vi "Initialize.vi"(8 "error in (no error)":errorcluster, 9 "Requestor":string, 10 "Requestee":string, 11 "RUS Measurement in":refnum<class "RUS Measurement.lvclass">) -> (0 "error out":errorcluster, 3 "RUS Measurement out":refnum<class "RUS Measurement.lvclass">)   [LabVIEW 2015, in "RUS Measurement.lvclass"]
uses:
  RUS Measurement.lvclass
  RUS Measurement.lvclass/RUS Measurement.ctl
  Write Active.vi
  Mag Lab Measurement/Mag Lab Measurement.lvclass
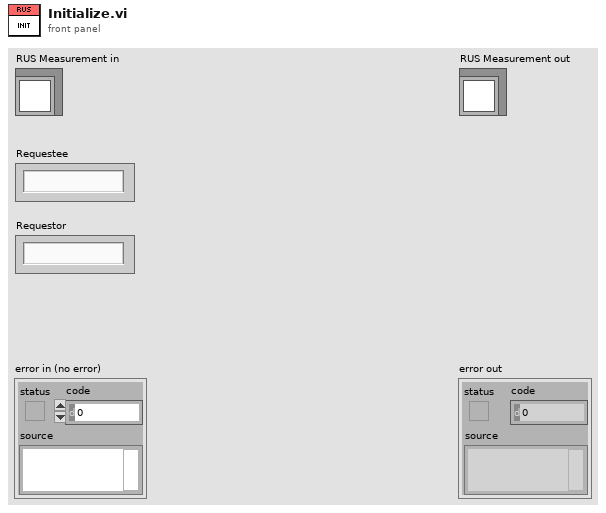
[diagram p1: front panel]
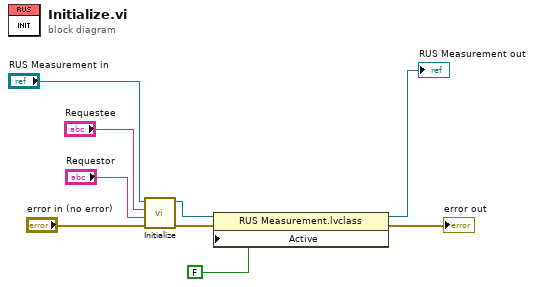
[diagram p0: block diagram]
diagram:
  n1 = call-parent "Initialize.vi"("error in (no error)"="error in (no error)", "Requestor"="Requestor", "Requestee"="Requestee", "Mag Lab Root in"="RUS Measurement in") -> ("error out"=w2:errorcluster, "Mag Lab Root out"=w5:refnum<class "RUS Measurement.lvclass">)  [unwired: 6 in]
  n2 = property class="RUS Measurement.lvclass"(reference=w5, error in=w2, "Active"=FALSE) -> (reference out=→"RUS Measurement out":refnum<class "RUS Measurement.lvclass">, error out=→"error out":errorcluster)
